vi "FM.vi"(0 "VISA session":refnum<visa-resource-name>, 1 "Dev (10.0 kHz)":dbl=10.0 min=0.0 max=2000.0 format="%.2f", 2 "State (F:Off)":bool=TRUE, 3 "State (F:Off)":bool, 4 "Dev (10.0kHz)":dbl=10.0 min=0.0 max=2000.0 format="%.2f", 5 "error in (no error)":errorcluster, 6 "PM1 Dev (1.0)":dbl=1.0 min=-360.0 max=360.0 format="%.2f", 7 "PM2 Dev (1.0)":dbl=1.0 min=-360.0 max=360.0 format="%.2f", 8 "Mod. Source (0:LFgen1)":i32(ring) items=["LFgen1", "External1", "External2"], 9 "Mod. Source (0:LFgen2)":i32(ring) items=["LFgen2", "External2"], 10 "LF Gen1 Freq (1:1kHz)":i16(ring)=1 items=["0.4kHz", "1kHz", "3kHz", "15kHz"], 11 "LFgen2 Freq (1kHz)":dbl=1.0 min=0.0001 max=2000.0 format="%.2f", 12 "FM/PM Mod (F:FM)":bool, 13 "LFgen2 Shape (0:Sinusoid)":i16(ring) items=["Sinusoid", "Square", "Triangle", "Noise", "Sawtooth"], 15 "Ext1 Coup (F:AC)":bool=TRUE, 16 "Ext2 Coup (F:AC)":bool=TRUE, 17 "Dev Unit PM (F:Rads)":bool, 18 "PM Bandwidth (0:100k)":i32(ring) items=["100kHz", "2MHz"]) -> (14 "dup VISA session":refnum<visa-resource-name>, 19 "error out":errorcluster)   [LabVIEW 2025]
doc: "Settings for frequency/phase modulation. The following modulation modes cannot be set simultaneously and disable each other: FM an PM; FM2/PM and STEREO; FM2/PM2 SOURCE = LFGEN2 and VOR, ILS, MKR BCN"
panel:
  # "Degrees\nRadians"
  # "PM\nFM"
  # "DC\nAC"
  # "DC\nAC"
  # "FM1/PM1"
  # "On\nOff"
  # "FM2/PM2"
  # "On\nOff"
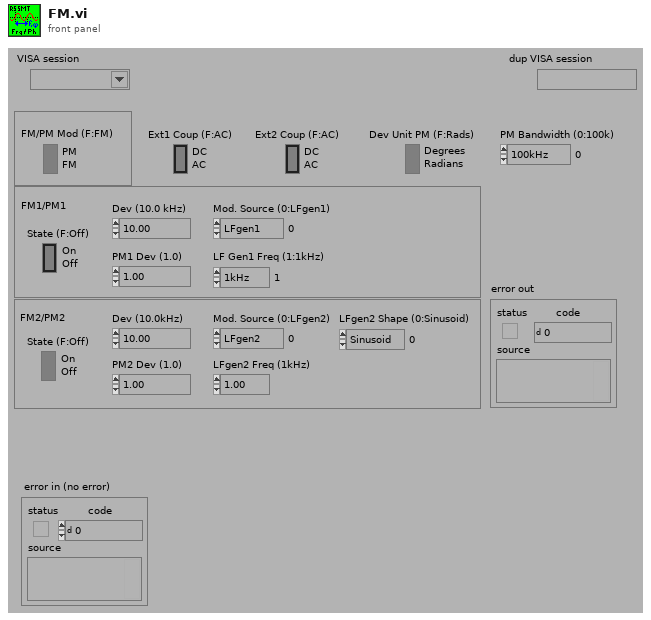
[diagram p1: front panel]
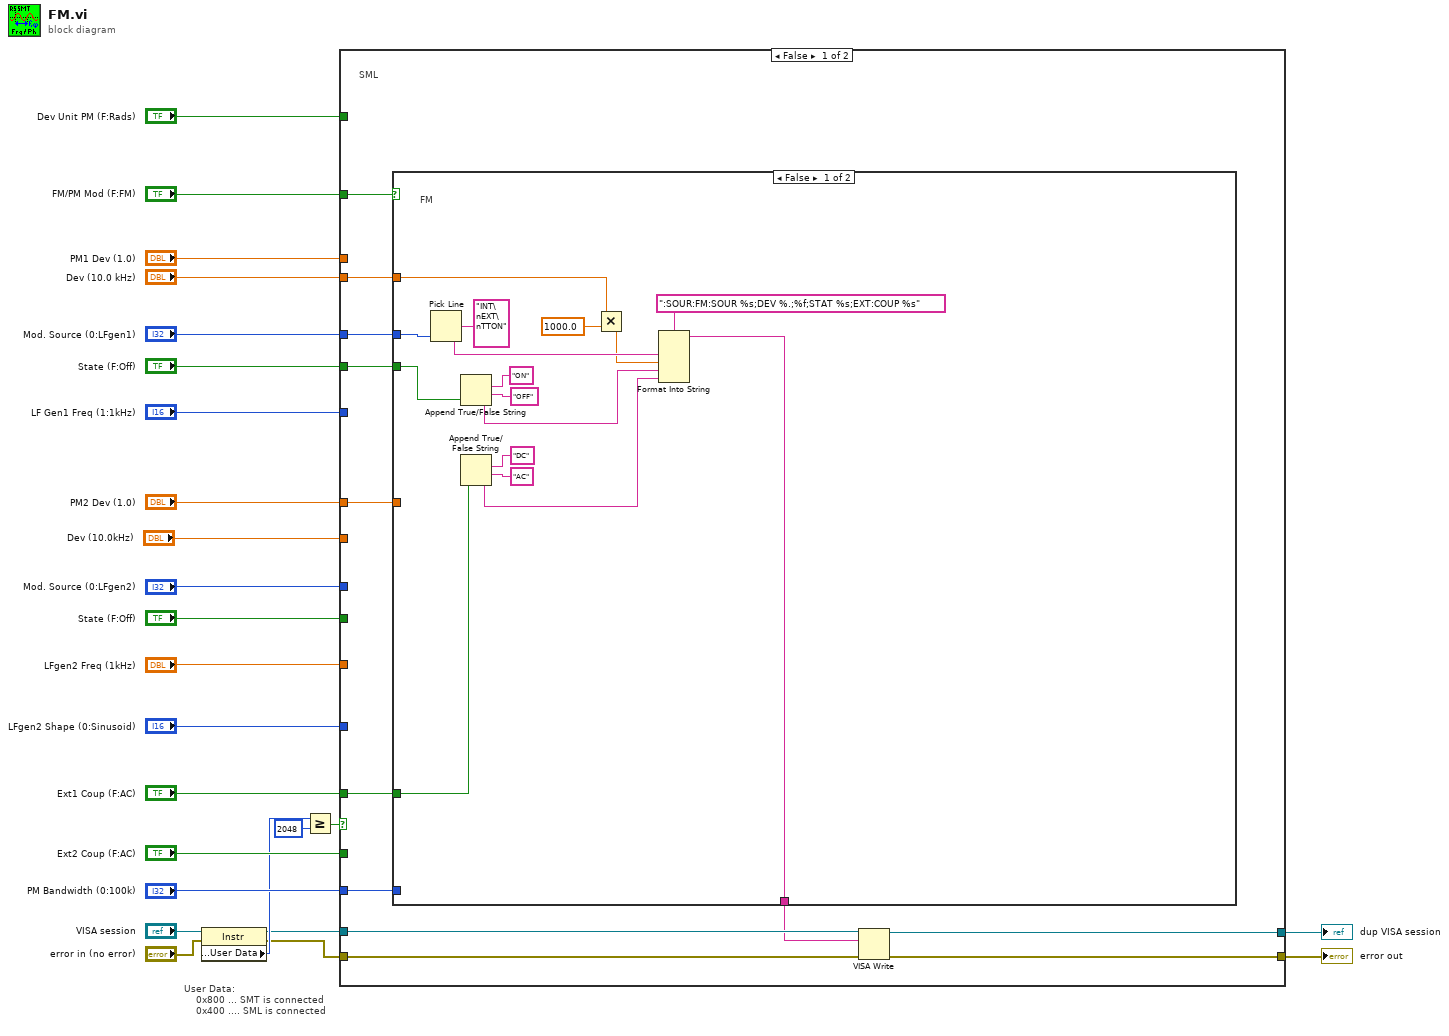
[diagram p0: block diagram]
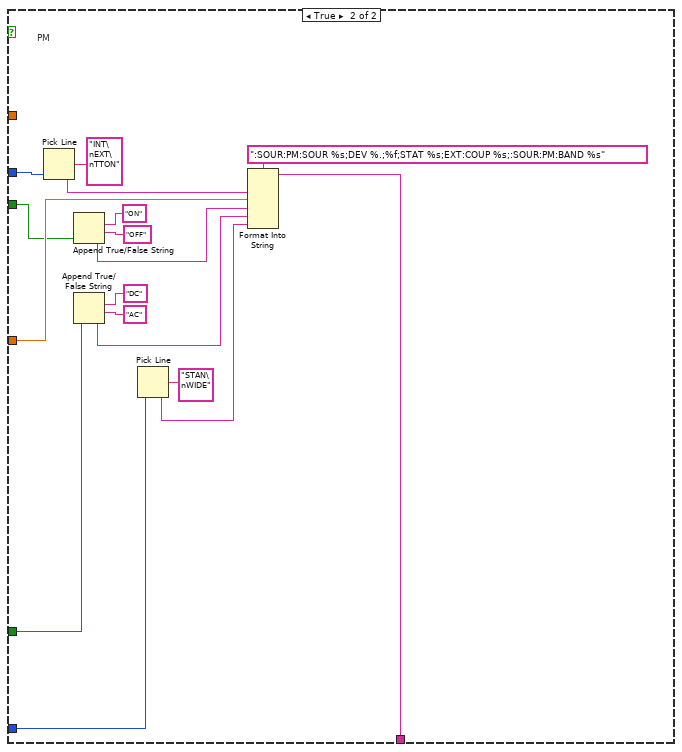
[diagram p2: hidden frame]
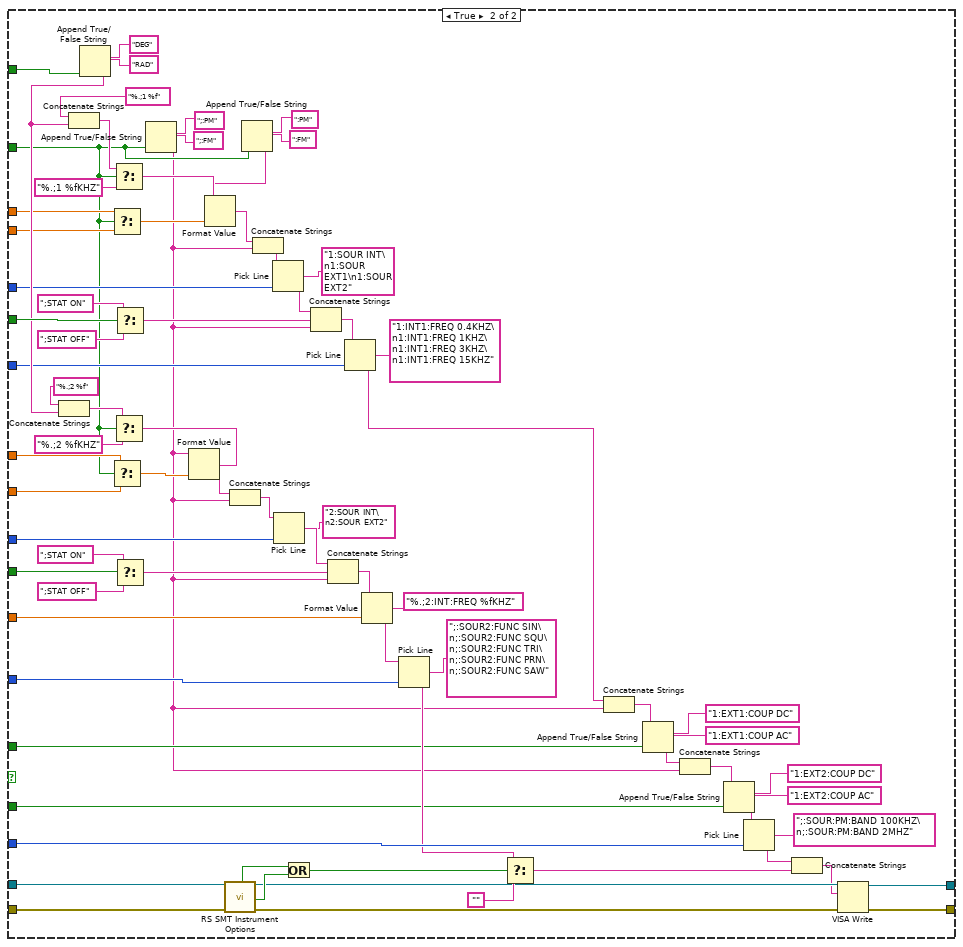
[diagram p3: hidden frame]
diagram:
  # "User Data:\n    0x800 ... SMT is connected\n    0x400 .... SML is connected"
  n1 = property class="Instr"(reference="VISA session", error in="error in (no error)") -> (reference out=w5:refnum<visa-resource-name>, error out=w4:errorcluster, "General Settings:User Data"=w7:u32)
  n2 = Greater Or Equal?(x=w7, y=u16 2048) -> (x >= y?=w1:bool)
  n3 = case shown="False" w1 {
    tunnel: "PM Bandwidth (0:100k)" -> [w26 w149]
    tunnel: w4 -> [w31 w139]
    tunnel: w5 -> [w32 w136]
    tunnel: "State (F:Off)" -> [_ w132]
    tunnel: "State (F:Off)" -> [w34 w125]
    tunnel: "Ext2 Coup (F:AC)" -> [_ w123]
    tunnel: "Ext1 Coup (F:AC)" -> [w33 w118]
    tunnel: "LFgen2 Shape (0:Sinusoid)" -> [_ w113]
    tunnel: "LFgen2 Freq (1kHz)" -> [_ w112]
    tunnel: "Mod. Source (0:LFgen2)" -> [_ w111]
    tunnel: "FM/PM Mod (F:FM)" -> [w37 w73]
    tunnel: "Dev (10.0kHz)" -> [_ w109]
    tunnel: "PM2 Dev (1.0)" -> [w27 w108]
    tunnel: "LF Gen1 Freq (1:1kHz)" -> [_ w97]
    tunnel: "Mod. Source (0:LFgen1)" -> [w36 w91]
    tunnel: "Dev Unit PM (F:Rads)" -> [_ w86]
    tunnel: "Dev (10.0 kHz)" -> [w35 w82]
    tunnel: "PM1 Dev (1.0)" -> [_ w81]
    tunnel: [w29 w77] -> w24
    tunnel: [w30 w76] -> w25
    frame False {
      # "SML"
      n4 = case shown="False" w37 {
        tunnel: w36 -> [w52 w61]
        tunnel: w35 -> [w47 _]
        tunnel: w34 -> [w44 w59]
        tunnel: w33 -> [w40 w58]
        tunnel: [w38 w54] -> w28
        tunnel: w27 -> [_ w60]
        tunnel: w26 -> [_ w57]
        frame False {
          # "FM"
          n5 = Pick Line(multi-line string="INT\nEXT\nTTON", line index=w52) -> (output string=w50:string)  [unwired: 1 in]
          n6 = Append True/False String(1:w44, 2:"OFF" ("false string"), 3:"ON" ("true string")) -> (0:w43:string)  [unwired: 1 in]
          n7 = Append True/False String(1:w40, 2:"AC" ("false string"), 3:"DC" ("true string")) -> (0:w39:string)  [unwired: 1 in]
          n8 = Multiply(x=w47, y=1000.0) -> (x*y=w45:dbl)
          n9 = Format Into String(format string=":SOUR:FM:SOUR %s;DEV %.;%f;STAT %s;EXT:COUP %s", w50, w45, w43, w39) -> (resulting string=w38:string)  [unwired: 2 in, 1 out]
        }
        frame True {
          # "PM"
          n10 = Pick Line(multi-line string="INT\nEXT\nTTON", line index=w61) -> (output string=w69:string)  [unwired: 1 in]
          n11 = Append True/False String(1:w59, 2:"OFF" ("false string"), 3:"ON" ("true string")) -> (0:w66:string)  [unwired: 1 in]
          n12 = Append True/False String(1:w58, 2:"AC" ("false string"), 3:"DC" ("true string")) -> (0:w63:string)  [unwired: 1 in]
          n13 = Pick Line(multi-line string="STAN\nWIDE", line index=w57) -> (output string=w55:string)  [unwired: 1 in]
          n14 = Format Into String(format string=":SOUR:PM:SOUR %s;DEV %.;%f;STAT %s;EXT:COUP %s;:SOUR:PM:BAND %s", w69, w60, w66, w63, w55) -> (resulting string=w54:string)  [unwired: 2 in, 1 out]
        }
      }
      n15 = VISA Write(VISA resource name=w32, write buffer=w28, error in (no error)=w31) -> (VISA resource name out=w30:refnum<visa-resource-name>, error out=w29:errorcluster)  [unwired: 1 out]
    }
    frame True {
      n16 = Append True/False String(1:w86, 2:"RAD", 3:"DEG") -> (0:w107:string)  [unwired: 1 in]
      n17 = Concatenate Strings("%.;2 %f", w107) -> (w101:string)
      n18 = Concatenate Strings("%.;1 %f", w107) -> (w90:string)
      n19 = Select(t=w81, s=w73, f=w82) -> (s? t:f=w83:dbl)
      n20 = Select(t=w108, s=w73, f=w109) -> (s? t:f=w99:dbl)
      n21 = Select(t=w90, s=w73, f="%.;1 %fKHZ") -> (s? t:f=w85:string)
      n22 = Select(t=w101, s=w73, f="%.;2 %fKHZ") -> (s? t:f=w110:string)
      n23 = Select(t=";STAT ON", s=w125, f=";STAT OFF") -> (s? t:f=w124:string)
      n24 = Select(t=";STAT ON", s=w132, f=";STAT OFF") -> (s? t:f=w131:string)
      n25 = Append True/False String(1:w73, 2:";:FM", 3:";:PM") -> (0:w72:string)  [unwired: 1 in]
      n26 = Format Value(string ("")=w72, format string=w110, value (0)=w99) -> (output string=w102:string)
      n27 = call "RS SMT Instrument Options.vi"("VISA session"=w136, "error in (no error)"=w139) -> ("3"=w145:bool, "dup VISA session"=w137:refnum<visa-resource-name>, "7"=w144:bool, "error out"=w138:errorcluster)  [unwired: 3 in, 11 out]
      n28 = Concatenate Strings(w102, w72) -> (w103:string)
      n29 = Append True/False String(1:w73, 2:":FM", 3:":PM") -> (0:w71:string)  [unwired: 1 in]
      n30 = Format Value(string ("")=w71, format string=w85, value (0)=w83) -> (output string=w92:string)
      n31 = Concatenate Strings(w92, w72) -> (w93:string)
      n32 = Pick Line(string ("")=w93, multi-line string="1:SOUR INT\n1:SOUR EXT1\n1:SOUR EXT2", line index=w91) -> (output string=w94:string)
      n33 = Pick Line(string ("")=w103, multi-line string="2:SOUR INT\n2:SOUR EXT2", line index=w111) -> (output string=w128:string)
      n34 = Or(x=w145, y=w144) -> (x .or. y?=w143:bool)
      n35 = Concatenate Strings(w94, w124, w72) -> (w95:string)
      n36 = Concatenate Strings(w128, w131, w72) -> (w104:string)
      n37 = Pick Line(string ("")=w95, multi-line string="1:INT1:FREQ 0.4KHZ\n1:INT1:FREQ 1KHZ\n1:INT1:FREQ 3KHZ\n1:INT1:FREQ 15KHZ", line index=w97) -> (output string=w135:string)
      n38 = Format Value(string ("")=w104, format string="%.;2:INT:FREQ %fKHZ", value (0)=w112) -> (output string=w133:string)
      n39 = Pick Line(string ("")=w133, multi-line string=";:SOUR2:FUNC SIN\n;:SOUR2:FUNC SQU\n;:SOUR2:FUNC TRI\n;:SOUR2:FUNC PRN\n;:SOUR2:FUNC SAW", line index=w113) -> (output string=w140:string)
      n40 = Select(t=w140, s=w143, f="") -> (s? t:f=w142:string)
      n41 = Concatenate Strings(w135, w72) -> (w117:string)
      n42 = Append True/False String(1:w118, 2:"1:EXT1:COUP AC", 3:"1:EXT1:COUP DC", 4:w117) -> (0:w120:string)
      n43 = Concatenate Strings(w120, w72) -> (w121:string)
      n44 = Append True/False String(1:w123, 2:"1:EXT2:COUP AC", 3:"1:EXT2:COUP DC", 4:w121) -> (0:w147:string)
      n45 = Pick Line(string ("")=w147, multi-line string=";:SOUR:PM:BAND 100KHZ\n;:SOUR:PM:BAND 2MHZ", line index=w149) -> (output string=w146:string)
      n46 = Concatenate Strings(w146, w142) -> (w134:string)
      n47 = VISA Write(VISA resource name=w137, write buffer=w134, error in (no error)=w138) -> (VISA resource name out=w76:refnum<visa-resource-name>, error out=w77:errorcluster)  [unwired: 1 out]
    }
  }
  "error out" <- w24
  "dup VISA session" <- w25
